vi "FPGALeftReadout.vi"() -> ()   [LabVIEW 2018]
uses:
  State.ctl
  PWMStates.ctl
  LightSensorStates.ctl
  Data.ctl
  <vilib>/rvi/Emulation/niFpgaGetClockAttributes.vi
  <vilib>/rvi/Emulation/niFpgaSctlEmulationGetInTimedLoop.vi
  <vilib>/rvi/Emulation/niFpgaEmulationReportErrorSimple.vi
  <vilib>/rvi/Emulation/niFpgaProcessEmulError.vi
  <vilib>/rvi/eio/common/nirviEmuTemplateMethod_errors.vi
  <vilib>/rvi/Emulation/niFpgaCriticalErrorInLSC.vi
  <vilib>/eio/EIONode/EIONode.xnode
panel:
  out "Boolean":bool
  out "Light Sensor State":T1
  out "Rotor Speed (Hz)":sgl
  in  "Motor debounce time (us)":u32=50
  out "ConnectorB/AI0":u16
  out "Motor read count":u64
  out "Motor half rev time (us)":u32
  out "Light Sensor":bool
  out "PWM State":T2
  in  "PWM Switch":bool
  in  "Pulse Width (us)":u32=1000 min=1000 max=2000
  in  "Frequency":i16=50 min=50 max=400
  in  "PowerDown? 3":bool
  out "Data 3":i32
  in  "Gain/ChannelSelect 3":T3(ring)
  out "ConnectorA/DIO4":bool
  out "State 3":T4
  out "Data array3":i32[](array[numeric])
  in  "PowerDown? 2":bool
  out "Data 2":i32
  in  "Gain/ChannelSelect 2":T3(ring)
  out "ConnectorA/DIO2":bool
  out "State 2":T4
  out "Data array 2":i32[](array[numeric])
  out "RawCurrent":u16
  out "RawVoltage":i16
  out "State":T4
  out "ConnectorA/DIO0":bool
  out "Data array":i32[](array[numeric])
  in  "PowerDown?":bool
  out "Data":i32
  in  "Gain/ChannelSelect":T3(ring)
  in  "stop":bool
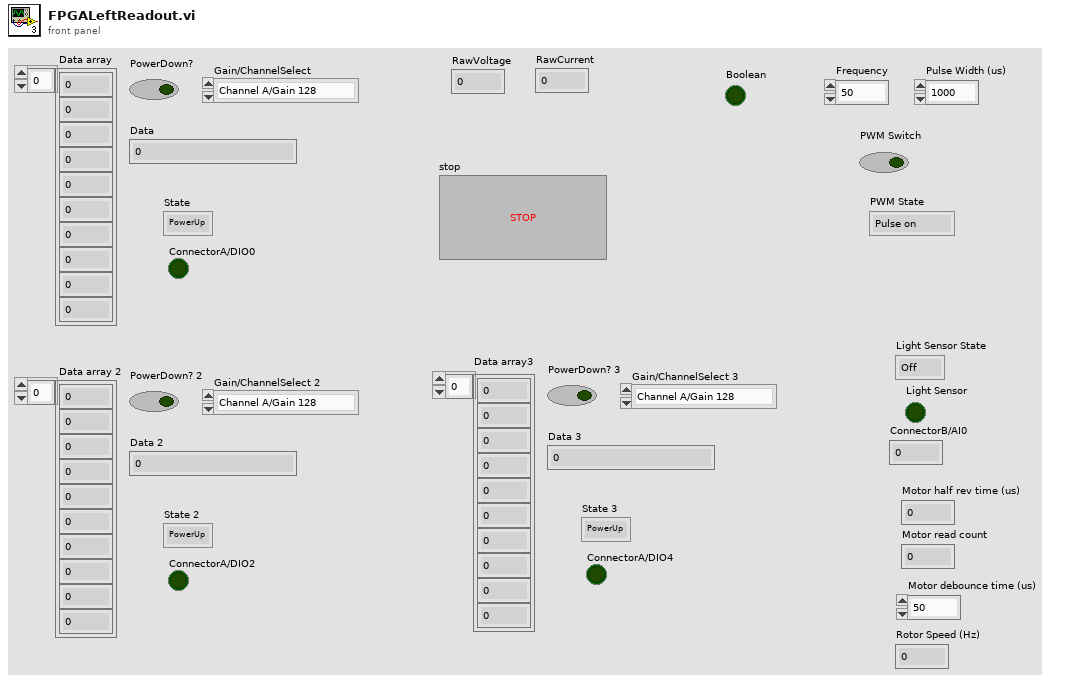
[diagram p1: front panel]
types:
  T1 = typedef "LightSensorStates.ctl" = enum16{"Off", "OffToOn", "On", "OnToOff"}
  T2 = typedef "PWMStates.ctl" = enum16{"Pulse on", "Hold pulse", "Pulse off", "Wait"}
  T3 = enum16{"Channel A/Gain 128", "Channel A/Gain 64", "Channel B/Gain 32"}
  T4 = typedef "State.ctl" = enum16{"PowerUp", "PowerDown", "Gain/ChannelSelect", "ReadData", "ClockLow", "ClockHigh", "ConvertData", "RetrievalReady?"}
  T5 = typedef "Data.ctl" = cluster{"DT":bool, "SCK":bool, "2's Data":i32, "PulseCount":u8, "DelayTime":u8, "Data":i32, "PowerDown?":bool, "Gain/ChannelSelect":enum16{"Channel A/Gain 128", "Channel A/Gain 64", "Channel B/Gain 32"}}
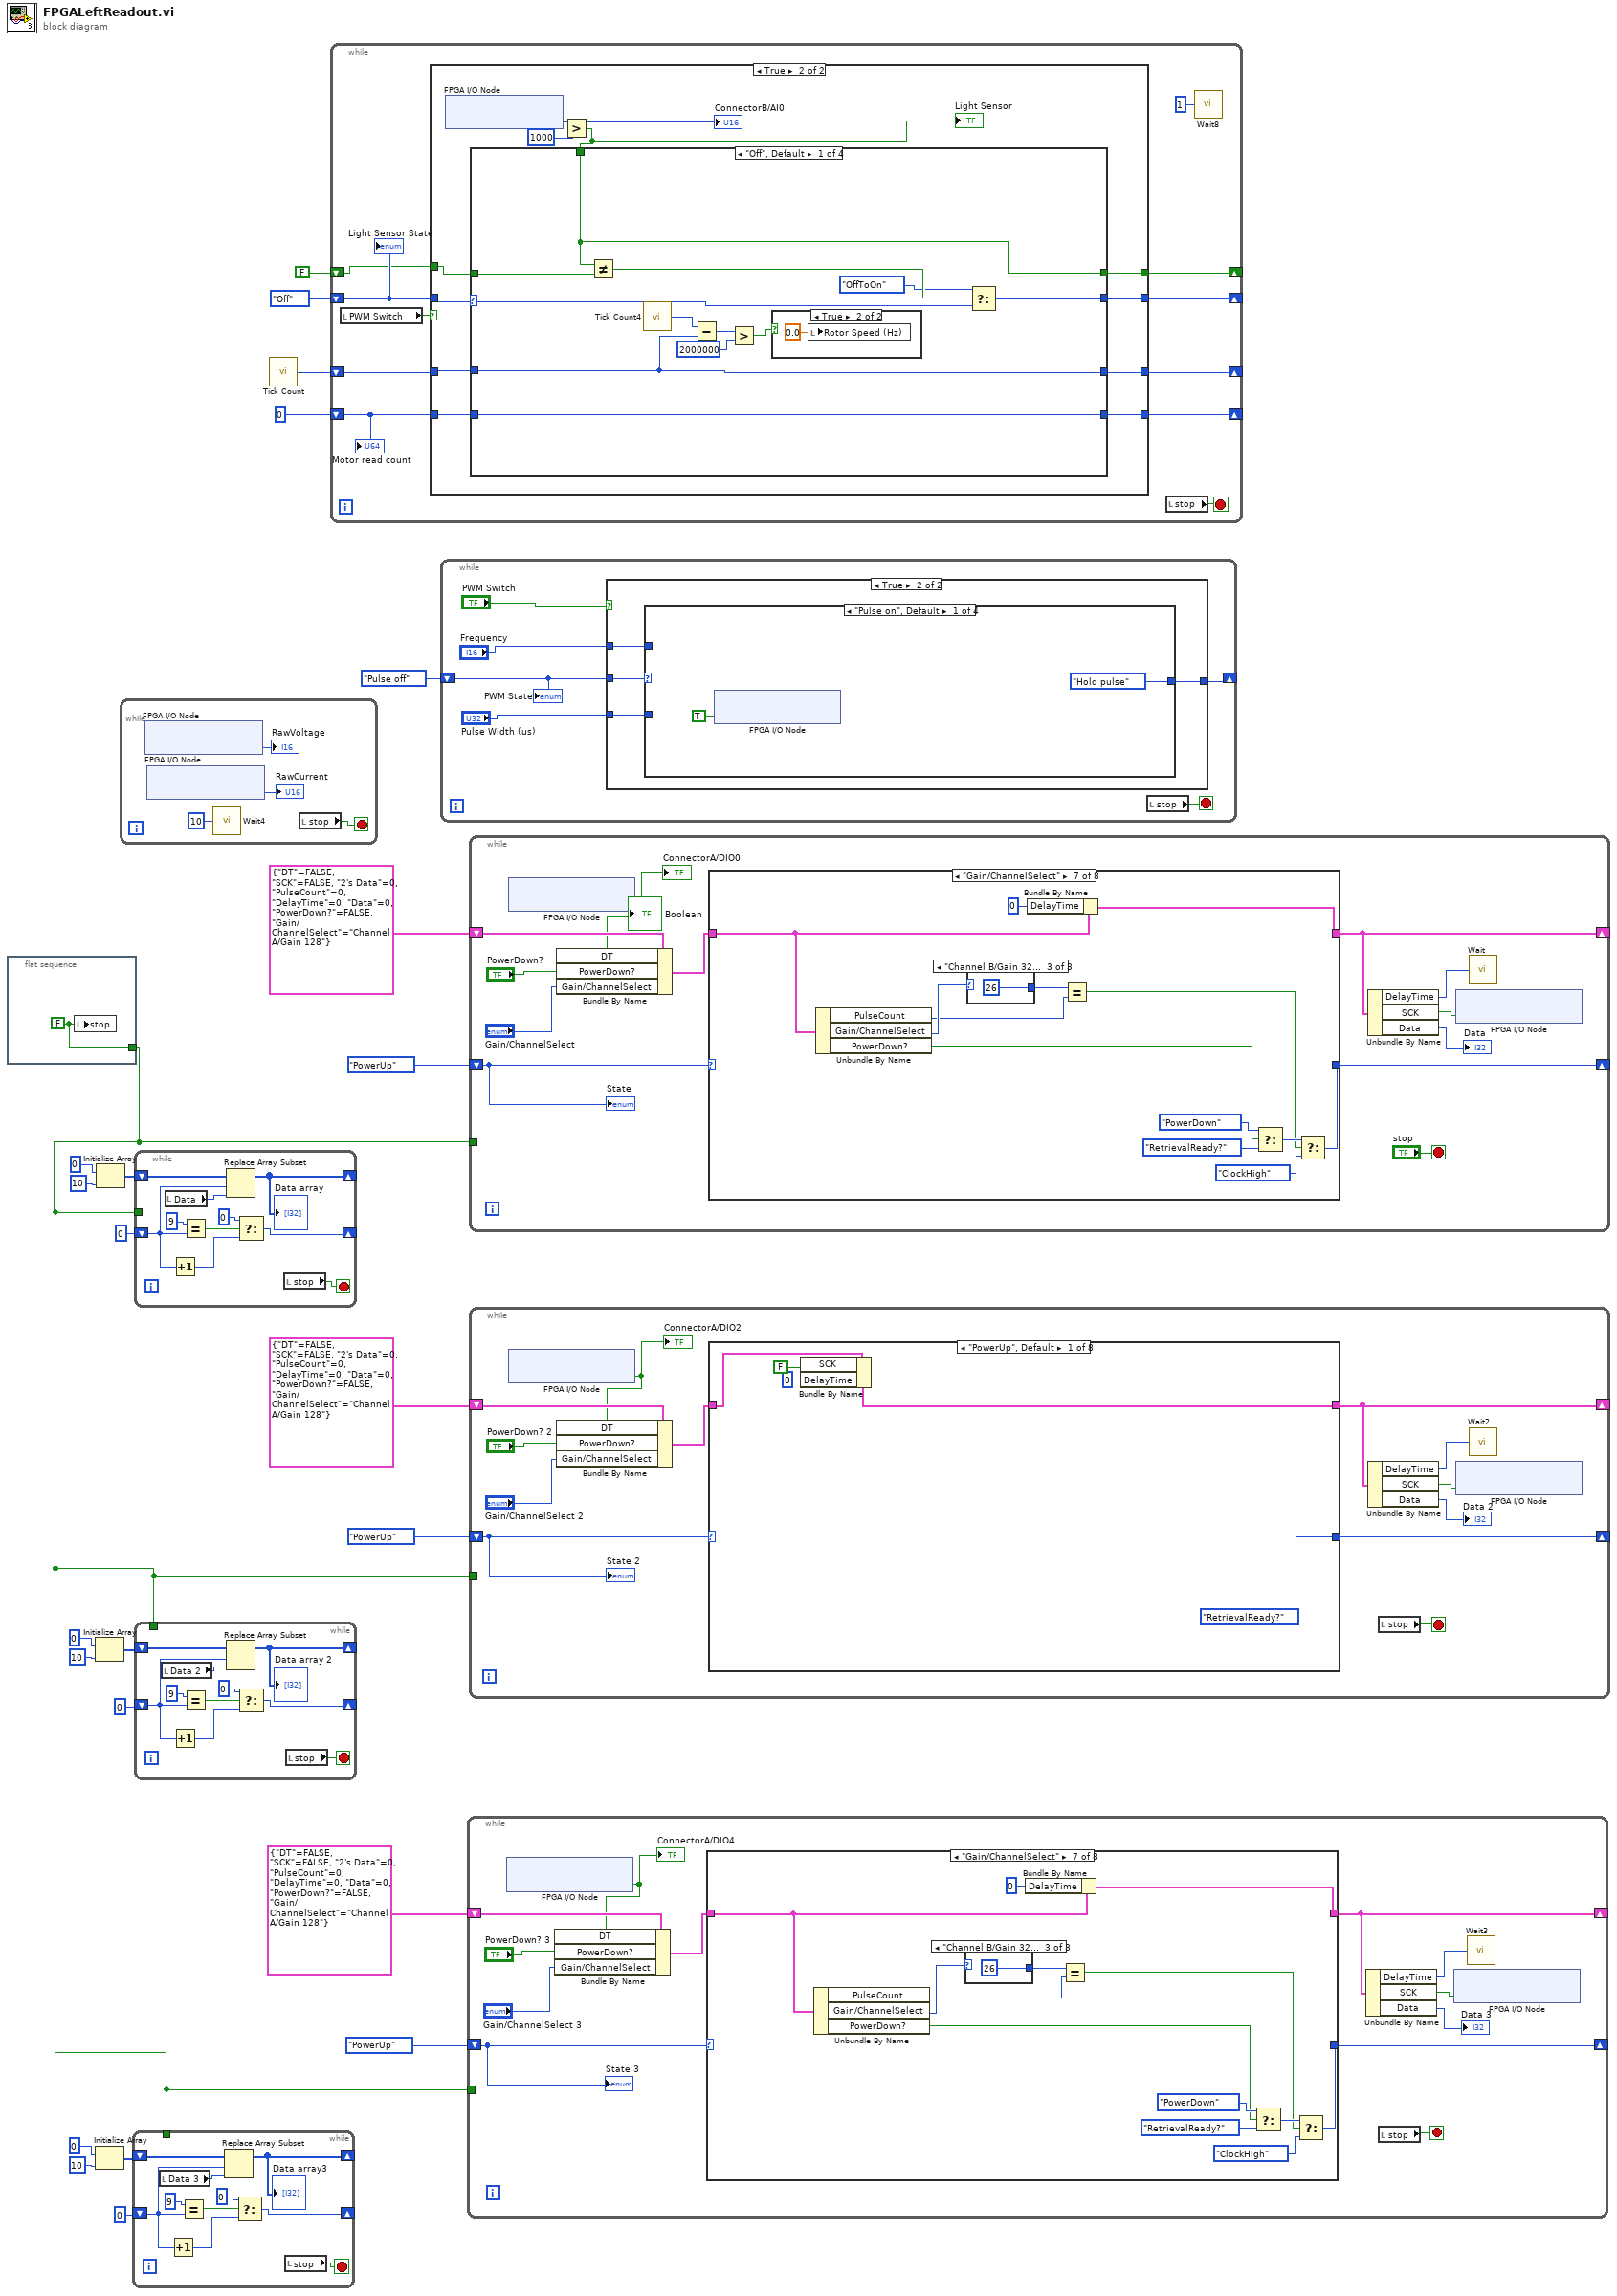
[diagram p0: block diagram]
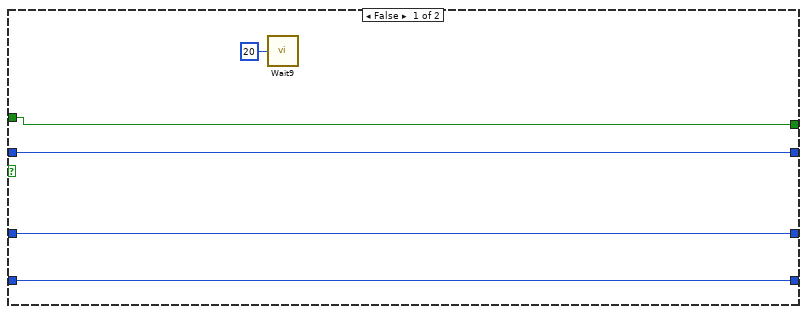
[diagram p2: hidden frame]
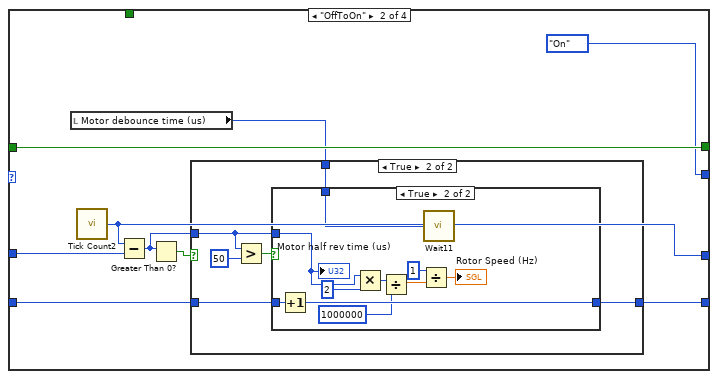
[diagram p4: hidden frame]
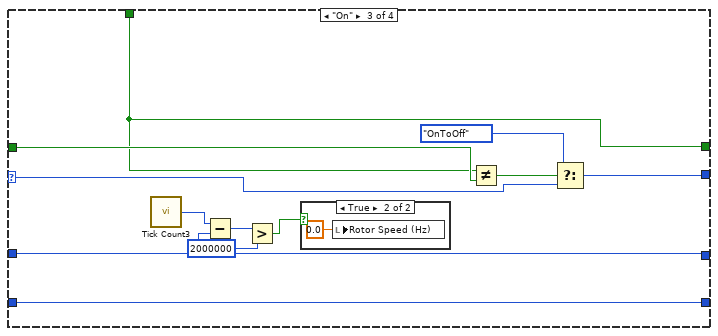
[diagram p7: hidden frame]
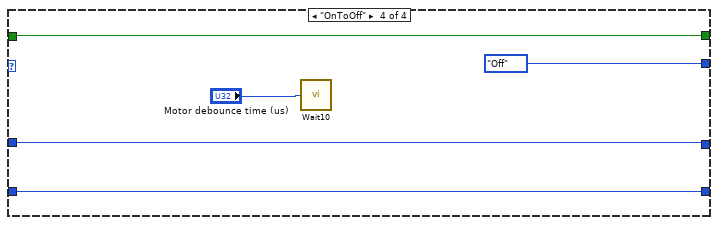
[diagram p9: hidden frame]
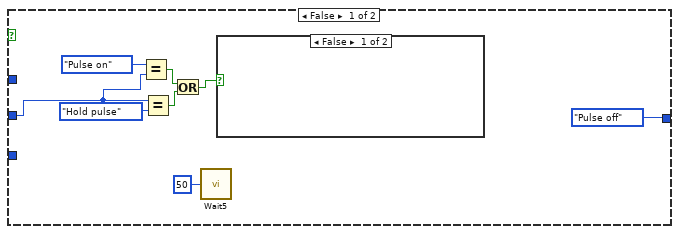
[diagram p10: hidden frame]
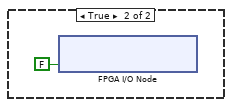
[diagram p11: hidden frame]
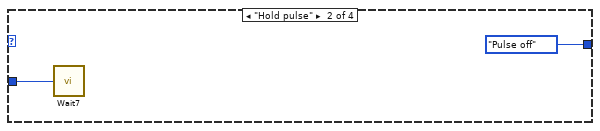
[diagram p12: hidden frame]
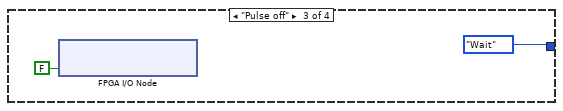
[diagram p13: hidden frame]
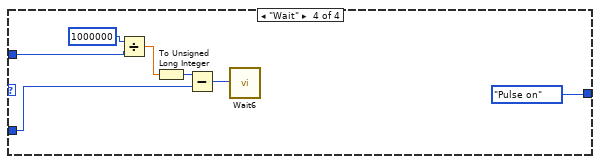
[diagram p14: hidden frame]
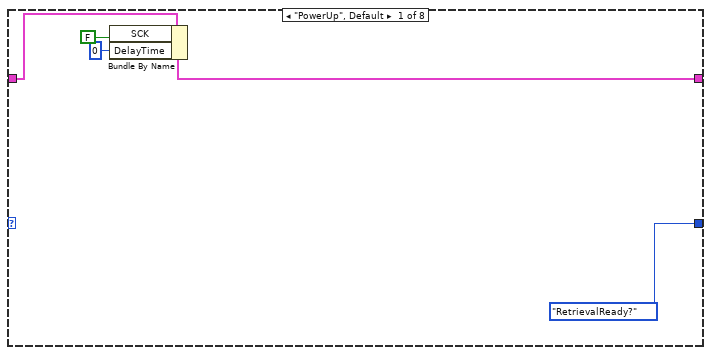
[diagram p15: hidden frame]
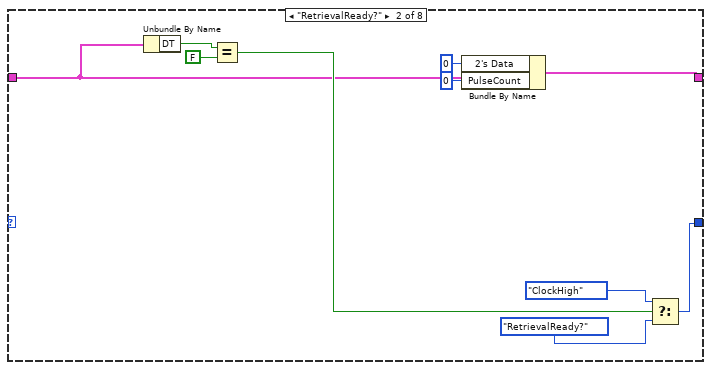
[diagram p16: hidden frame]
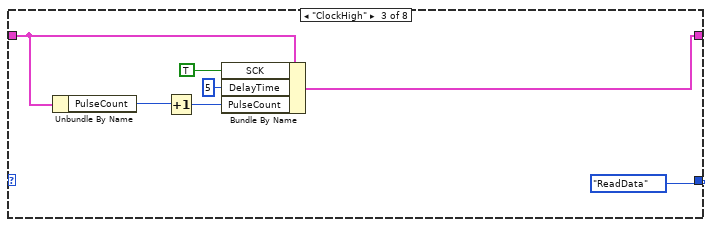
[diagram p17: hidden frame]
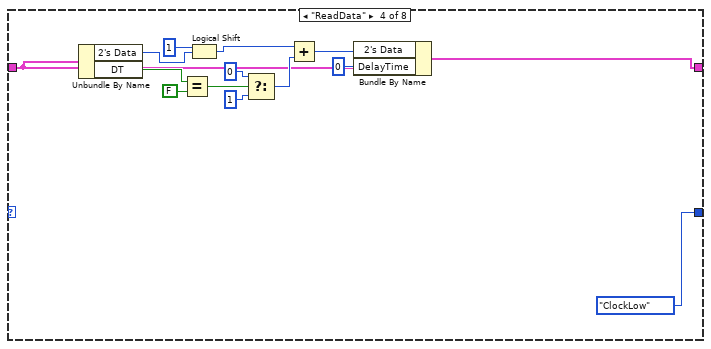
[diagram p18: hidden frame]
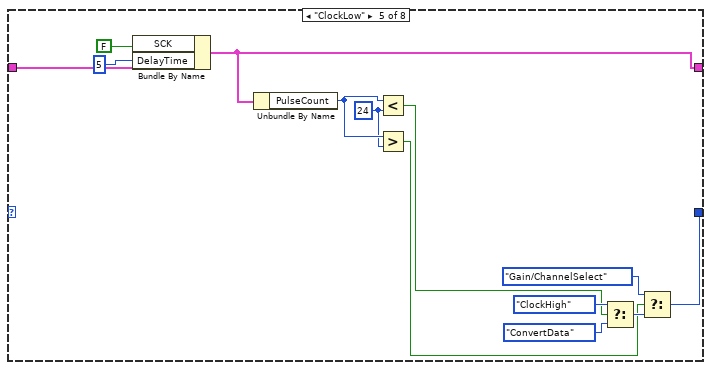
[diagram p19: hidden frame]
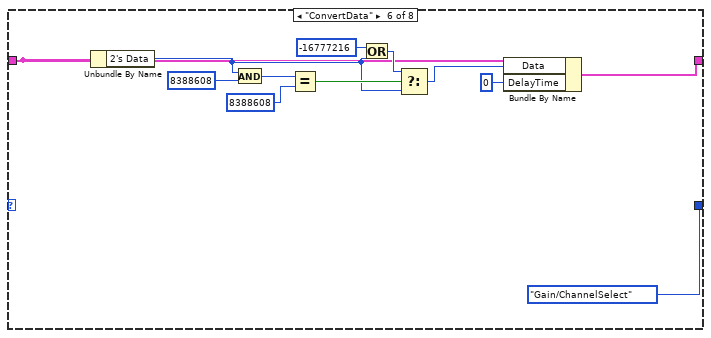
[diagram p20: hidden frame]
diagram:
  n1 = flat-sequence {
    tunnel: [w25] -> w14
    frame #0 {
      w25 = FALSE
      n2 = local write "stop"(w25) -> ()
    }
  }
  n3 = Initialize Array(0 ("Data"), 10 ("dimension size")) -> (w10:i32[])
  n4 = Initialize Array(0 ("Data"), 10 ("dimension size")) -> (w7:i32[])
  n5 = Initialize Array(0 ("Data"), 10 ("dimension size")) -> (w21:i32[])
  n6 = while {
    stop <- w27 stop-if-true
    n7 = xnode "FPGA I/O Node"() -> ("ConnectorC/AI0"=→"RawVoltage":i16)  [unwired: 1 in, 1 out]
    n8 = xnode "FPGA I/O Node"() -> ("ConnectorA/AI0"=→"RawCurrent":u16)  [unwired: 1 in, 1 out]
    n9 = call "Wait4"("Count(mSec)"=u32 10) -> ()  [unwired: 1 out]
    n10 = local read "stop"() -> (w27:bool)
  }
  n11 = while {
    shift-right: [w31] -> _
    shift-left: w7 -> [w32]
    shift-right: [w37] -> _
    shift-left: 0 ("index") -> [w33]
    tunnel: w14 -> [_]
    stop <- w30 stop-if-true
    n12 = local read "Data 3"() -> (w39:i32)
    n13 = Increment(x=w33) -> (x+1=w36:i32)
    n14 = Equal?(x=9, y=w33) -> (x = y?=w34:bool)
    n15 = Replace Array Subset(array=w32, new element=w39, index=w33) -> (w31:i32[])
    "Data array3" <- w31
    n16 = Select(t=0 ("index"), s=w34, f=w36) -> (s? t:f=w37:i32)
    n17 = local read "stop"() -> (w30:bool)
  }
  n18 = while {
    shift-right: [w41] -> _
    shift-left: w21 -> [w42]
    shift-right: [w47] -> _
    shift-left: 0 ("index") -> [w43]
    tunnel: w14 -> [_]
    stop <- w40 stop-if-true
    n19 = local read "Data"() -> (w49:i32)
    n20 = Increment(x=w43) -> (x+1=w46:i32)
    n21 = Equal?(x=9, y=w43) -> (x = y?=w44:bool)
    n22 = Replace Array Subset(array=w42, new element=w49, index=w43) -> (w41:i32[])
    "Data array" <- w41
    n23 = Select(t=0 ("index"), s=w44, f=w46) -> (s? t:f=w47:i32)
    n24 = local read "stop"() -> (w40:bool)
  }
  n25 = while {
    shift-right: [w51] -> _
    shift-left: w10 -> [w52]
    shift-right: [w57] -> _
    shift-left: 0 ("index") -> [w53]
    tunnel: w14 -> [_]
    stop <- w50 stop-if-true
    n26 = local read "Data 2"() -> (w59:i32)
    n27 = Increment(x=w53) -> (x+1=w56:i32)
    n28 = Equal?(x=9, y=w53) -> (x = y?=w54:bool)
    n29 = Replace Array Subset(array=w52, new element=w59, index=w53) -> (w51:i32[])
    "Data array 2" <- w51
    n30 = Select(t=0 ("index"), s=w54, f=w56) -> (s? t:f=w57:i32)
    n31 = local read "stop"() -> (w50:bool)
  }
  n32 = call "Tick Count"() -> ("Tick Count(uSec)"=w3:u32)
  n33 = while {
    shift-right: [w63] -> _
    shift-left: FALSE -> [w64]
    shift-right: [w66] -> _
    shift-left: w3 -> [w69]
    shift-right: [w65] -> _
    shift-left: LightSensorStates."Off" -> [w67]
    shift-right: [w61] -> _
    shift-left: u64 0 -> [w62]
    stop <- w70 stop-if-true
    n34 = local read "PWM Switch"() -> (w68:bool)
    n35 = case shown="True" w68 {
      tunnel: w69 -> [w74 w83]
      tunnel: w67 -> [w73 w86]
      tunnel: [w74 w79] -> w66
      tunnel: [w73 w82] -> w65
      tunnel: w64 -> [w72 w85]
      tunnel: [w72 w84] -> w63
      tunnel: w62 -> [w71 w81]
      tunnel: [w71 w80] -> w61
      frame False {
        n36 = call "Wait9"("Count(mSec)"=u32 20 ("Count(uSec)")) -> ()  [unwired: 1 out]
      }
      frame True {
        n37 = xnode "FPGA I/O Node"() -> ("ConnectorB/AI0"=w78:u16)  [unwired: 1 in, 1 out]
        "ConnectorB/AI0" <- w78
        n38 = Greater?(x=w78, y=u16 1000) -> (0:w76:bool)
        "Light Sensor" <- w76
        n39 = case shown="\"Off\", Default" w86 {
          selector: w86 -> [w94 _ w134 _]
          tunnel: w85 -> [w98 w106 w136 w143]
          tunnel: [w97 w106 w135 w143] -> w84
          tunnel: w76 -> [w97 _ w135 _]
          tunnel: w83 -> [w88 w108 w131 w142]
          tunnel: [w92 LightSensorStates."On" w138 LightSensorStates."Off"] -> w82
          tunnel: w81 -> [w93 w104 w132 w141]
          tunnel: [w93 w103 w132 w141] -> w80
          tunnel: [w88 w102 w131 w142] -> w79
          frame "Off", Default {
            n40 = Not Equal?(x=w97, y=w98) -> (x != y?=w96:bool)
            n41 = call "Tick Count4"() -> ("Tick Count(uSec)"=w91:u32)
            n42 = Subtract(x=w91, y=w88) -> (x-y=w90:u32)
            n43 = Greater?(x=w90, y=u32 2000000) -> (0:w87:bool)
            n44 = case shown="True" w87 {
              frame False {
              }
              frame True {
                n45 = local write "Rotor Speed (Hz)"(sgl 0.0 ("Rotor Speed (Hz)")) -> ()
              }
            }
            n46 = Select(t=LightSensorStates."OffToOn", s=w96, f=w94) -> (s? t:f=w92:T1)
          }
          frame "OffToOn" {
            n47 = local read "Motor debounce time (us)"() -> (w101:u32)
            n48 = call "Tick Count2"() -> ("Tick Count(uSec)"=w102:u32)
            n49 = Subtract(x=w102, y=w108) -> (x-y=w105:u32)
            n50 = Greater Than 0?(x=w105) -> (x > 0?=w107:bool)
            n51 = case shown="True" w107 {
              tunnel: w105 -> [_ w112]
              tunnel: w104 -> [w109 w115]
              tunnel: [w109 w114] -> w103
              tunnel: w101 -> [_ w110]
              frame False {
              }
              frame True {
                n52 = Greater?(x=w112, y=u32 50) -> (0:w113:bool)
                n53 = case shown="True" w113 {
                  tunnel: w112 -> [_ w123]
                  tunnel: w115 -> [w116 w126]
                  tunnel: [w116 w125] -> w114
                  tunnel: w110 -> [_ w124]
                  frame False {
                  }
                  frame True {
                    n54 = Increment(x=w126) -> (x+1=w125:u64)
                    n55 = Multiply(x=w123, y=u32 2) -> (x*y=w121:u32)
                    n56 = Divide(x=w121, y=u32 1000000) -> (x/y=w118:sgl)
                    n57 = Divide(x=i16 1, y=w118) -> (x/y=→"Rotor Speed (Hz)":sgl)
                    n58 = call "Wait11"("Count(uSec)"=w124) -> ()  [unwired: 1 out]
                    "Motor half rev time (us)" <- w123
                  }
                }
              }
            }
          }
          frame "On" {
            n59 = call "Tick Count3"() -> ("Tick Count(uSec)"=w130:u32)
            n60 = Subtract(x=w130, y=w131) -> (x-y=w129:u32)
            n61 = Greater?(x=w129, y=u32 2000000) -> (0:w127:bool)
            n62 = case shown="True" w127 {
              frame False {
              }
              frame True {
                n63 = local write "Rotor Speed (Hz)"(sgl 0.0 ("Rotor Speed (Hz)")) -> ()
              }
            }
            n64 = Not Equal?(x=w135, y=w136) -> (x != y?=w137:bool)
            n65 = Select(t=LightSensorStates."OnToOff", s=w137, f=w134) -> (s? t:f=w138:T1)
          }
          frame "OnToOff" {
            n66 = call "Wait10"("Count(uSec)"="Motor debounce time (us)") -> ()  [unwired: 1 out]
          }
        }
      }
    }
    n67 = local read "stop"() -> (w70:bool)
    n68 = call "Wait8"("Count(uSec)"=u32 1) -> ()  [unwired: 1 out]
    "Motor read count" <- w62
    "Light Sensor State" <- w67
  }
  n69 = while {
    shift-right: [w145] -> _
    shift-left: PWMStates."Pulse off" -> [w150]
    stop <- w149 stop-if-true
    n70 = case shown="True" "PWM Switch" {
      tunnel: w150 -> [w154 w163]
      tunnel: "Pulse Width (us)" -> [_ w162]
      tunnel: "Frequency" -> [_ w161]
      tunnel: [PWMStates."Pulse off" w160] -> w145
      frame False {
        n71 = Equal?(x=PWMStates."Pulse on", y=w154) -> (x = y?=w152:bool)
        n72 = Equal?(x=w154, y=PWMStates."Hold pulse") -> (x = y?=w151:bool)
        n73 = Or(x=w152, y=w151) -> (x .or. y?=w153:bool)
        n74 = call "Wait5"("Count(mSec)"=u32 50) -> ()  [unwired: 1 out]
        n75 = case shown="False" w153 {
          frame False {
          }
          frame True {
            n76 = xnode "FPGA I/O Node"("ConnectorA/DIO8"=FALSE) -> ()  [unwired: 1 in, 1 out]
          }
        }
      }
      frame True {
        n77 = case shown="\"Pulse on\", Default" w163 {
          tunnel: w162 -> [_ w167 _ w175]
          tunnel: w161 -> [_ _ _ w171]
          tunnel: [PWMStates."Hold pulse" PWMStates."Pulse off" PWMStates."Wait" PWMStates."Pulse on"] -> w160
          frame "Pulse on", Default {
            n78 = xnode "FPGA I/O Node"("ConnectorA/DIO8"=TRUE) -> ()  [unwired: 1 in, 1 out]
          }
          frame "Hold pulse" {
            n79 = call "Wait7"("Count(uSec)"=w167) -> ()  [unwired: 1 out]
          }
          frame "Pulse off" {
            n80 = xnode "FPGA I/O Node"("ConnectorA/DIO8"=FALSE) -> ()  [unwired: 1 in, 1 out]
          }
          frame "Wait" {
            n81 = Divide(x=u32 1000000 ("y"), y=w171) -> (x/y=w170:sgl)
            n82 = To Unsigned Long Integer(number=w170) -> (unsigned 32bit integer=w176:u32)
            n83 = Subtract(x=w176, y=w175) -> (x-y=w174:u32)
            n84 = call "Wait6"("Count(uSec)"=w174) -> ()  [unwired: 1 out]
          }
        }
      }
    }
    n85 = local read "stop"() -> (w149:bool)
    "PWM State" <- w150
  }
  n86 = while {
    shift-right: [w180] -> _
    shift-left: T5 {"DT"=FALSE, "SCK"=FALSE, "2's Data"=0, "PulseCount"=0, "DelayTime"=0, "Data"=0, "PowerDown?"=FALSE, "Gain/ChannelSelect"=enum."Channel A/Gain 128"} ("Data") -> [w185]
    shift-right: [w186] -> _
    shift-left: State."PowerUp" ("State") -> [w188]
    tunnel: w14 -> [_]
    stop <- w177 stop-if-true
    n87 = xnode "FPGA I/O Node"() -> ("ConnectorA/DIO4"=w183:bool)  [unwired: 1 in, 1 out]
    "ConnectorA/DIO4" <- w183
    n88 = Bundle By Name(cluster=w185, "DT"=w183, "PowerDown?"="PowerDown? 3", "Gain/ChannelSelect"="Gain/ChannelSelect 3") -> (w184:T5)
    n89 = case shown="\"Gain/ChannelSelect\"" w188 {
      tunnel: w184 -> [w193 w197 w206 w211 w237 w242 w252 w267]
      tunnel: [w191 w196 w210 w213 w232 w241 w251 w273] -> w180
      tunnel: [State."RetrievalReady?" ("State") w199 State."ReadData" ("State") State."ClockLow" ("State") w233 State."Gain/ChannelSelect" ("State") w259 w268] -> w186
      frame "PowerUp", Default {
        n90 = Bundle By Name(cluster=w193, "SCK"=FALSE, "DelayTime"=u8 0) -> (w191:T5)
      }
      frame "RetrievalReady?" {
        n91 = Unbundle By Name(w197) -> ("DT"=w203:bool)
        n92 = Equal?(x=w203, y=FALSE) -> (x = y?=w198:bool)
        n93 = Bundle By Name(cluster=w197, "2's Data"=0, "PulseCount"=u8 0) -> (w196:T5)
        n94 = Select(t=State."ClockHigh" ("State"), s=w198, f=State."RetrievalReady?" ("State")) -> (s? t:f=w199:T4)
      }
      frame "ClockHigh" {
        n95 = Unbundle By Name(w206) -> ("PulseCount"=w205:u8)
        n96 = Increment(x=w205) -> (x+1=w204:u8)
        n97 = Bundle By Name(cluster=w206, "SCK"=TRUE, "DelayTime"=u8 5, "PulseCount"=w204) -> (w210:T5)
      }
      frame "ReadData" {
        n98 = Unbundle By Name(w211) -> ("2's Data"=w224:i32, "DT"=w222:bool)
        n99 = Equal?(x=w222, y=FALSE ("SCK")) -> (x = y?=w220:bool)
        n100 = Logical Shift(y=i16 1, x=w224) -> (x << y=w219:i32)
        n101 = Select(t=0 ("DelayTime"), s=w220, f=1 ("DelayTime")) -> (s? t:f=w216:i32)
        n102 = Add(x=w219, y=w216) -> (x+y=w215:i32)
        n103 = Bundle By Name(cluster=w211, "2's Data"=w215, "DelayTime"=u8 0) -> (w213:T5)
      }
      frame "ClockLow" {
        w226 = u8 24 ("y")
        n104 = Bundle By Name(cluster=w237, "SCK"=FALSE, "DelayTime"=u8 5) -> (w232:T5)
        n105 = Unbundle By Name(w232) -> ("PulseCount"=w227:u8)
        n106 = Less?(x=w227, y=w226) -> (x < y?=w229:bool)
        n107 = Greater?(x=w227, y=w226) -> (0:w225:bool)
        n108 = Select(t=State."ClockHigh" ("State"), s=w229, f=State."ConvertData" ("State")) -> (s? t:f=w228:T4)
        n109 = Select(t=State."Gain/ChannelSelect" ("State"), s=w225, f=w228) -> (s? t:f=w233:T4)
      }
      frame "ConvertData" {
        n110 = Unbundle By Name(w242) -> ("2's Data"=w243:i32)
        n111 = And(x=w243, y=8388608) -> (x .and. y?=w248:i32)
        n112 = Equal?(x=w248, y=8388608) -> (x = y?=w246:bool)
        n113 = Or(x=-16777216 ("y"), y=w243) -> (x .or. y?=w244:i32)
        n114 = Select(t=w244, s=w246, f=w243) -> (s? t:f=w239:i32)
        n115 = Bundle By Name(cluster=w242, "Data"=w239, "DelayTime"=u8 0) -> (w241:T5)
      }
      frame "Gain/ChannelSelect" {
        n116 = Unbundle By Name(w252) -> ("PulseCount"=w255:u8, "Gain/ChannelSelect"=w257:T3, "PowerDown?"=w258:bool)
        n117 = case shown="\"Channel B/Gain 32\"" w257 {
          tunnel: [u8 25 ("PulseCount") u8 27 ("PulseCount") u8 26 ("PulseCount")] -> w256
          frame "Channel A/Gain 128", Default {
          }
          frame "Channel A/Gain 64" {
          }
          frame "Channel B/Gain 32" {
          }
        }
        n118 = Bundle By Name(cluster=w252, "DelayTime"=u8 0) -> (w251:T5)
        n119 = Equal?(x=w256, y=w255) -> (x = y?=w253:bool)
        n120 = Select(t=State."PowerDown" ("State"), s=w258, f=State."RetrievalReady?" ("State")) -> (s? t:f=w254:T4)
        n121 = Select(t=w254, s=w253, f=State."ClockHigh" ("State")) -> (s? t:f=w259:T4)
      }
      frame "PowerDown" {
        n122 = Unbundle By Name(w267) -> ("PowerDown?"=w266:bool)
        n123 = Bundle By Name(cluster=w267, "SCK"=TRUE, "DelayTime"=u8 70) -> (w273:T5)
        n124 = Select(t=State."PowerDown" ("State"), s=w266, f=State."PowerUp" ("State")) -> (s? t:f=w268:T4)
      }
    }
    n125 = Unbundle By Name(w180) -> ("DelayTime"=w187:u8, "SCK"=w179:bool, "Data"=→"Data 3":i32)
    n126 = local read "stop"() -> (w177:bool)
    n127 = xnode "FPGA I/O Node"("ConnectorA/DIO5"=w179) -> ()  [unwired: 1 in, 1 out]
    n128 = call "Wait3"("Count(uSec)"=w187) -> ()  [unwired: 1 out]
    "State 3" <- w188
  }
  n129 = while {
    shift-right: [w276] -> _
    shift-left: T5 {"DT"=FALSE, "SCK"=FALSE, "2's Data"=0, "PulseCount"=0, "DelayTime"=0, "Data"=0, "PowerDown?"=FALSE, "Gain/ChannelSelect"=enum."Channel A/Gain 128"} ("Data") -> [w282]
    shift-right: [w283] -> _
    shift-left: State."PowerUp" ("State") -> [w285]
    tunnel: w14 -> [_]
    stop <- "stop" stop-if-true
    n130 = xnode "FPGA I/O Node"() -> ("ConnectorA/DIO0"=w280:bool)  [unwired: 1 in, 1 out]
    "ConnectorA/DIO0" <- w280
    n131 = Bundle By Name(cluster=w282, "DT"=w280, "PowerDown?"="PowerDown?", "Gain/ChannelSelect"="Gain/ChannelSelect") -> (w281:T5)
    n132 = case shown="\"Gain/ChannelSelect\"" w285 {
      tunnel: w281 -> [w290 w294 w303 w308 w334 w339 w349 w364]
      tunnel: [w288 w293 w307 w310 w329 w338 w348 w370] -> w276
      tunnel: [State."RetrievalReady?" ("State") w296 State."ReadData" ("State") State."ClockLow" ("State") w330 State."Gain/ChannelSelect" ("State") w356 w365] -> w283
      frame "PowerUp", Default {
        n133 = Bundle By Name(cluster=w290, "SCK"=FALSE, "DelayTime"=u8 0) -> (w288:T5)
      }
      frame "RetrievalReady?" {
        n134 = Unbundle By Name(w294) -> ("DT"=w300:bool)
        n135 = Equal?(x=w300, y=FALSE) -> (x = y?=w295:bool)
        n136 = Bundle By Name(cluster=w294, "2's Data"=0, "PulseCount"=u8 0) -> (w293:T5)
        n137 = Select(t=State."ClockHigh" ("State"), s=w295, f=State."RetrievalReady?" ("State")) -> (s? t:f=w296:T4)
      }
      frame "ClockHigh" {
        n138 = Unbundle By Name(w303) -> ("PulseCount"=w302:u8)
        n139 = Increment(x=w302) -> (x+1=w301:u8)
        n140 = Bundle By Name(cluster=w303, "SCK"=TRUE, "DelayTime"=u8 5, "PulseCount"=w301) -> (w307:T5)
      }
      frame "ReadData" {
        n141 = Unbundle By Name(w308) -> ("2's Data"=w321:i32, "DT"=w319:bool)
        n142 = Equal?(x=w319, y=FALSE ("SCK")) -> (x = y?=w317:bool)
        n143 = Logical Shift(y=i16 1, x=w321) -> (x << y=w316:i32)
        n144 = Select(t=0 ("DelayTime"), s=w317, f=1 ("DelayTime")) -> (s? t:f=w313:i32)
        n145 = Add(x=w316, y=w313) -> (x+y=w312:i32)
        n146 = Bundle By Name(cluster=w308, "2's Data"=w312, "DelayTime"=u8 0) -> (w310:T5)
      }
      frame "ClockLow" {
        w323 = u8 24 ("y")
        n147 = Bundle By Name(cluster=w334, "SCK"=FALSE, "DelayTime"=u8 5) -> (w329:T5)
        n148 = Unbundle By Name(w329) -> ("PulseCount"=w324:u8)
        n149 = Less?(x=w324, y=w323) -> (x < y?=w326:bool)
        n150 = Greater?(x=w324, y=w323) -> (0:w322:bool)
        n151 = Select(t=State."ClockHigh" ("State"), s=w326, f=State."ConvertData" ("State")) -> (s? t:f=w325:T4)
        n152 = Select(t=State."Gain/ChannelSelect" ("State"), s=w322, f=w325) -> (s? t:f=w330:T4)
      }
      frame "ConvertData" {
        n153 = Unbundle By Name(w339) -> ("2's Data"=w340:i32)
        n154 = And(x=w340, y=8388608) -> (x .and. y?=w345:i32)
        n155 = Equal?(x=w345, y=8388608) -> (x = y?=w343:bool)
        n156 = Or(x=-16777216 ("y"), y=w340) -> (x .or. y?=w341:i32)
        n157 = Select(t=w341, s=w343, f=w340) -> (s? t:f=w336:i32)
        n158 = Bundle By Name(cluster=w339, "Data"=w336, "DelayTime"=u8 0) -> (w338:T5)
      }
      frame "Gain/ChannelSelect" {
        n159 = Unbundle By Name(w349) -> ("PulseCount"=w352:u8, "Gain/ChannelSelect"=w354:T3, "PowerDown?"=w355:bool)
        n160 = case shown="\"Channel B/Gain 32\"" w354 {
          tunnel: [u8 25 ("PulseCount") u8 27 ("PulseCount") u8 26 ("PulseCount")] -> w353
          frame "Channel A/Gain 128", Default {
          }
          frame "Channel A/Gain 64" {
          }
          frame "Channel B/Gain 32" {
          }
        }
        n161 = Bundle By Name(cluster=w349, "DelayTime"=u8 0) -> (w348:T5)
        n162 = Equal?(x=w353, y=w352) -> (x = y?=w350:bool)
        n163 = Select(t=State."PowerDown" ("State"), s=w355, f=State."RetrievalReady?" ("State")) -> (s? t:f=w351:T4)
        n164 = Select(t=w351, s=w350, f=State."ClockHigh" ("State")) -> (s? t:f=w356:T4)
      }
      frame "PowerDown" {
        n165 = Unbundle By Name(w364) -> ("PowerDown?"=w363:bool)
        n166 = Bundle By Name(cluster=w364, "SCK"=TRUE, "DelayTime"=u8 70) -> (w370:T5)
        n167 = Select(t=State."PowerDown" ("State"), s=w363, f=State."PowerUp" ("State")) -> (s? t:f=w365:T4)
      }
    }
    n168 = Unbundle By Name(w276) -> ("DelayTime"=w284:u8, "SCK"=w275:bool, "Data"=→"Data":i32)
    n169 = xnode "FPGA I/O Node"("ConnectorA/DIO1"=w275) -> ()  [unwired: 1 in, 1 out]
    n170 = call "Wait"("Count(uSec)"=w284) -> ()  [unwired: 1 out]
    "State" <- w285
  }
  n171 = while {
    shift-right: [w374] -> _
    shift-left: T5 {"DT"=FALSE, "SCK"=FALSE, "2's Data"=0, "PulseCount"=0, "DelayTime"=0, "Data"=0, "PowerDown?"=FALSE, "Gain/ChannelSelect"=enum."Channel A/Gain 128"} ("Data") -> [w379]
    shift-right: [w380] -> _
    shift-left: State."PowerUp" ("State") -> [w382]
    tunnel: w14 -> [_]
    stop <- w371 stop-if-true
    n172 = xnode "FPGA I/O Node"() -> ("ConnectorA/DIO2"=w377:bool)  [unwired: 1 in, 1 out]
    "ConnectorA/DIO2" <- w377
    n173 = Bundle By Name(cluster=w379, "DT"=w377, "PowerDown?"="PowerDown? 2", "Gain/ChannelSelect"="Gain/ChannelSelect 2") -> (w378:T5)
    n174 = case shown="\"PowerUp\", Default" w382 {
      tunnel: w378 -> [w387 w391 w400 w405 w431 w436 w446 w461]
      tunnel: [w385 w390 w404 w407 w426 w435 w445 w467] -> w374
      tunnel: [State."RetrievalReady?" ("State") w393 State."ReadData" ("State") State."ClockLow" ("State") w427 State."Gain/ChannelSelect" ("State") w453 w462] -> w380
      frame "PowerUp", Default {
        n175 = Bundle By Name(cluster=w387, "SCK"=FALSE, "DelayTime"=u8 0) -> (w385:T5)
      }
      frame "RetrievalReady?" {
        n176 = Unbundle By Name(w391) -> ("DT"=w397:bool)
        n177 = Equal?(x=w397, y=FALSE) -> (x = y?=w392:bool)
        n178 = Bundle By Name(cluster=w391, "2's Data"=0, "PulseCount"=u8 0) -> (w390:T5)
        n179 = Select(t=State."ClockHigh" ("State"), s=w392, f=State."RetrievalReady?" ("State")) -> (s? t:f=w393:T4)
      }
      frame "ClockHigh" {
        n180 = Unbundle By Name(w400) -> ("PulseCount"=w399:u8)
        n181 = Increment(x=w399) -> (x+1=w398:u8)
        n182 = Bundle By Name(cluster=w400, "SCK"=TRUE, "DelayTime"=u8 5, "PulseCount"=w398) -> (w404:T5)
      }
      frame "ReadData" {
        n183 = Unbundle By Name(w405) -> ("2's Data"=w418:i32, "DT"=w416:bool)
        n184 = Equal?(x=w416, y=FALSE ("SCK")) -> (x = y?=w414:bool)
        n185 = Logical Shift(y=i16 1, x=w418) -> (x << y=w413:i32)
        n186 = Select(t=0 ("DelayTime"), s=w414, f=1 ("DelayTime")) -> (s? t:f=w410:i32)
        n187 = Add(x=w413, y=w410) -> (x+y=w409:i32)
        n188 = Bundle By Name(cluster=w405, "2's Data"=w409, "DelayTime"=u8 0) -> (w407:T5)
      }
      frame "ClockLow" {
        w420 = u8 24 ("y")
        n189 = Bundle By Name(cluster=w431, "SCK"=FALSE, "DelayTime"=u8 5) -> (w426:T5)
        n190 = Unbundle By Name(w426) -> ("PulseCount"=w421:u8)
        n191 = Less?(x=w421, y=w420) -> (x < y?=w423:bool)
        n192 = Greater?(x=w421, y=w420) -> (0:w419:bool)
        n193 = Select(t=State."ClockHigh" ("State"), s=w423, f=State."ConvertData" ("State")) -> (s? t:f=w422:T4)
        n194 = Select(t=State."Gain/ChannelSelect" ("State"), s=w419, f=w422) -> (s? t:f=w427:T4)
      }
      frame "ConvertData" {
        n195 = Unbundle By Name(w436) -> ("2's Data"=w437:i32)
        n196 = And(x=w437, y=8388608) -> (x .and. y?=w442:i32)
        n197 = Equal?(x=w442, y=8388608) -> (x = y?=w440:bool)
        n198 = Or(x=-16777216 ("y"), y=w437) -> (x .or. y?=w438:i32)
        n199 = Select(t=w438, s=w440, f=w437) -> (s? t:f=w433:i32)
        n200 = Bundle By Name(cluster=w436, "Data"=w433, "DelayTime"=u8 0) -> (w435:T5)
      }
      frame "Gain/ChannelSelect" {
        n201 = Unbundle By Name(w446) -> ("PulseCount"=w449:u8, "Gain/ChannelSelect"=w451:T3, "PowerDown?"=w452:bool)
        n202 = case shown="\"Channel B/Gain 32\"" w451 {
          tunnel: [u8 25 ("PulseCount") u8 27 ("PulseCount") u8 26 ("PulseCount")] -> w450
          frame "Channel A/Gain 128", Default {
          }
          frame "Channel A/Gain 64" {
          }
          frame "Channel B/Gain 32" {
          }
        }
        n203 = Bundle By Name(cluster=w446, "DelayTime"=u8 0) -> (w445:T5)
        n204 = Equal?(x=w450, y=w449) -> (x = y?=w447:bool)
        n205 = Select(t=State."PowerDown" ("State"), s=w452, f=State."RetrievalReady?" ("State")) -> (s? t:f=w448:T4)
        n206 = Select(t=w448, s=w447, f=State."ClockHigh" ("State")) -> (s? t:f=w453:T4)
      }
      frame "PowerDown" {
        n207 = Unbundle By Name(w461) -> ("PowerDown?"=w460:bool)
        n208 = Bundle By Name(cluster=w461, "SCK"=TRUE, "DelayTime"=u8 70) -> (w467:T5)
        n209 = Select(t=State."PowerDown" ("State"), s=w460, f=State."PowerUp" ("State")) -> (s? t:f=w462:T4)
      }
    }
    n210 = Unbundle By Name(w374) -> ("DelayTime"=w381:u8, "SCK"=w373:bool, "Data"=→"Data 2":i32)
    n211 = local read "stop"() -> (w371:bool)
    n212 = xnode "FPGA I/O Node"("ConnectorA/DIO3"=w373) -> ()  [unwired: 1 in, 1 out]
    n213 = call "Wait2"("Count(uSec)"=w381) -> ()  [unwired: 1 out]
    "State 2" <- w382
  }
